vi "ErrorLog_LogError.vi"(8 "error in (no error)":errorcluster, 9 "Context (\"Error\")":string="Error", 10 "Error To Log":errorcluster, 11 "reference in":refnum<class "ErrorLog.lvclass">) -> (0 "error out":errorcluster, 1 "Error String":string, 2 "Cleaned Error":errorcluster, 3 "reference out":refnum<class "ErrorLog.lvclass">, 4 "Error was Logged":bool)   [LabVIEW 2014, in "ErrorLog.lvclass"]
uses:
  ErrorLog.lvclass
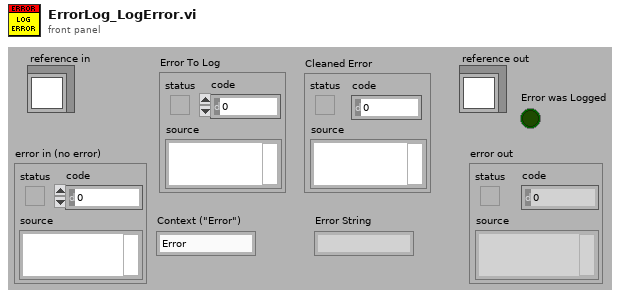
[diagram p1: front panel]
types:
  T1 = typedef "ErrorLog.lvclass/ObjectAttributes.ctl" = cluster{"ErrorFile":path, "Supress Consecutive Duplicates":bool, "Errors":string, "Quit":bool, "Errors since last call":string, "Last Recorded Error":string, "ErrorPath":path, "PossiblePaths":path[], "BaseFileName":string, "Max Log Files":i32, "ErrorFile Index":i32, "Max File Size":i64}
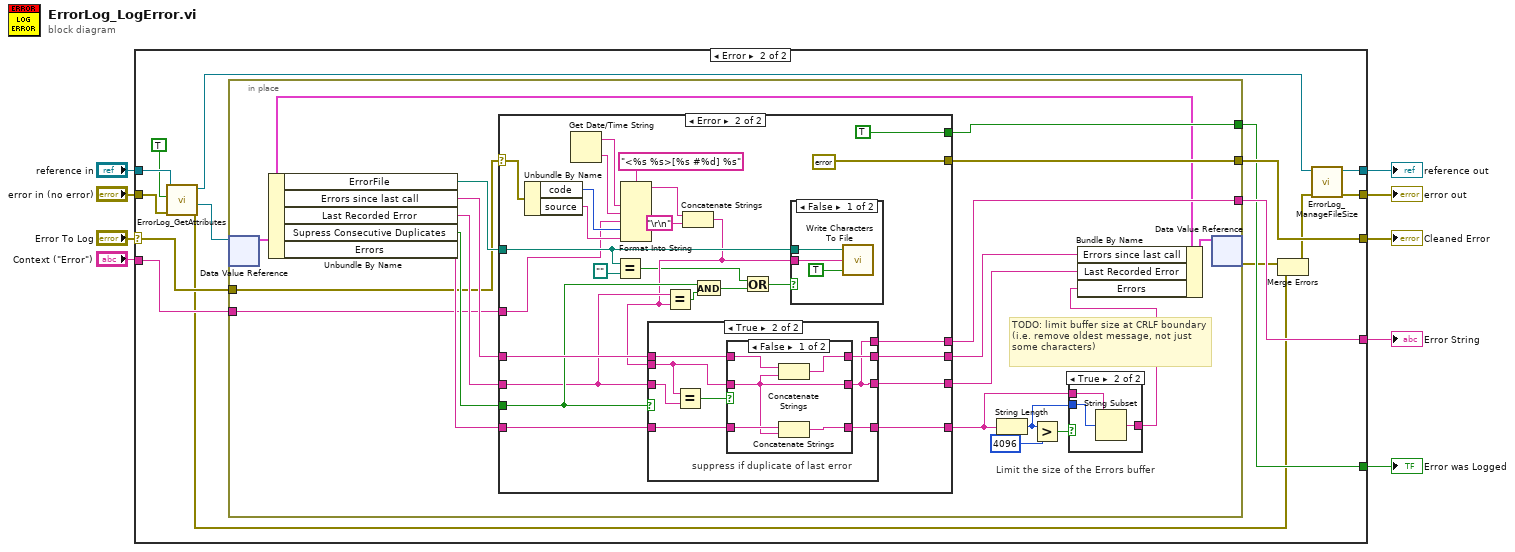
[diagram p0: block diagram]
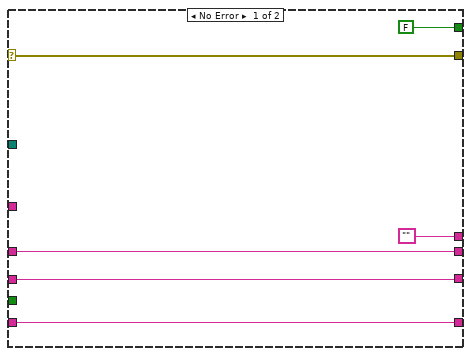
[diagram p4: hidden frame]
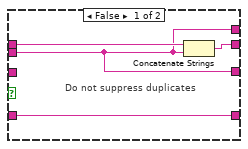
[diagram p6: hidden frame]
diagram:
  n1 = case shown="Error" "Error To Log" {
    selector: "Error To Log" -> [w11 w19]
    tunnel: [w11 w15] -> w9
    tunnel: [w10 w12] -> w7
    tunnel: "reference in" -> [w10 w26]
    tunnel: [_ w21] -> w6
    tunnel: [_ w23] -> w5
    tunnel: "error in (no error)" -> [_ w25]
    tunnel: "Context (\"Error\")" -> [_ w18]
    tunnel: [_ w22] -> w1
    frame No Error {
    }
    frame Error {
      n2 = call "ErrorLog_GetAttributes.vi"("error in (no error)"=w25, "OnlyGetDvrReference(False)"=TRUE, "reference in"=w26) -> ("error out"=w16:errorcluster, "DataRef"=w20:refnum<data-value>, "reference out"=w13:refnum<class "ErrorLog.lvclass">)  [unwired: 5 in, 1 out]
      n3 = in-place {
        in-place-border: [w33] -> w23
        in-place-border: [w32] -> w22
        in-place-border: [w31] -> w21
        in-place-border: w19 -> [w28]
        in-place-border: w18 -> [w27]
        # "TODO: limit buffer size at CRLF boundary (i.e. remove oldest message, not just some characters)"
        # "Limit the size of the Errors buffer"
        n4 = in-place-dvr #1(w20) -> (w30:T1)  [unwired: 1 out]
        n5 = Unbundle By Name(w30) -> ("ErrorFile"=w45:path, "Errors since last call"=w44:string, "Last Recorded Error"=w43:string, "Supress Consecutive Duplicates"=w42:bool, "Errors"=w39:string)
        n6 = case shown="Error" w28 {
          selector: w28 -> [w55 w80]
          tunnel: [w55 errorcluster {"status"=FALSE, "code"=0, "source"=""} ("error out")] -> w33
          tunnel: w45 -> [_ w67]
          tunnel: w44 -> [w54 w72]
          tunnel: [w54 w71] -> w40
          tunnel: w43 -> [w53 w64]
          tunnel: w42 -> [_ w65]
          tunnel: [w53 w70] -> w41
          tunnel: ["" w69] -> w32
          tunnel: [FALSE TRUE] -> w31
          tunnel: w39 -> [w50 w58]
          tunnel: [w50 w57] -> w35
          tunnel: w27 -> [_ w56]
          frame No Error {
          }
          frame Error {
            n7 = Unbundle By Name(w80) -> ("code"=w75:i32, "source"=w76:string)
            n8 = Get Date/Time String() -> (date string=w73:string, time string=w74:string)  [unwired: 3 in]
            n9 = Equal?(x=w67, y=path "") -> (x = y?=w61:bool)
            n10 = Format Into String(format string="<%s %s>[%s #%d] %s", w73, w74, w56, w75, w76) -> (resulting string=w77:string)  [unwired: 2 in, 1 out]
            n11 = Concatenate Strings(w77, "\r\n") -> (w63:string)
            n12 = case shown="True" w65 {
              tunnel: w72 -> [w88 w94]
              tunnel: w63 -> [w86 w92]
              tunnel: [w87 w93] -> w71
              tunnel: w64 -> [_ w95]
              tunnel: [w86 w91] -> w70
              tunnel: [w86 w91] -> w69
              tunnel: w58 -> [w85 w90]
              tunnel: [w85 w89] -> w57
              frame False {
                # "Do not suppress duplicates"
                n13 = Concatenate Strings(w88, w86) -> (w87:string)
              }
              frame True {
                # "suppress if duplicate of last error"
                n14 = Equal?(x=w92, y=w95) -> (x = y?=w96:bool)
                n15 = case shown="False" w96 {
                  tunnel: w92 -> [w98 w103]
                  tunnel: w94 -> [w101 w104]
                  tunnel: [w100 w104] -> w93
                  tunnel: [w98 w103] -> w91
                  tunnel: w90 -> [w99 w102]
                  tunnel: [w97 w102] -> w89
                  frame False {
                    n16 = Concatenate Strings(w101, w98) -> (w100:string)
                    n17 = Concatenate Strings(w99, w98) -> (w97:string)
                  }
                  frame True {
                    # "do not record again"
                  }
                }
              }
            }
            n18 = Equal?(x=w64, y=w63) -> (x = y?=w66:bool)
            n19 = And(x=w65, y=w66) -> (x .and. y?=w62:bool)
            n20 = Or(x=w61, y=w62) -> (x .or. y?=w60:bool)
            n21 = case shown="False" w60 {
              tunnel: w63 -> [w83 _]
              tunnel: w67 -> [w82 _]
              frame False {
                n22 = call <vilib>:"Write Characters To File.vi"("append to file? (new file:F)"=TRUE, "character string"=w83, "file path (dialog if empty)"=w82) -> ()  [unwired: 2 in, 1 out]
              }
              frame True {
                # "Object may already be destroyed"
                # "No File or suppressed"
              }
            }
          }
        }
        n23 = String Length(string=w35) -> (length=w36:i32)
        n24 = Greater?(x=w36, y=4096) -> (0:w37:bool)
        n25 = case shown="True" w37 {
          tunnel: w36 -> [_ w49]
          tunnel: w35 -> [w46 w48]
          tunnel: [w46 w47] -> w34
          frame False {
          }
          frame True {
            n26 = String Subset(string=w48, offset (0)=w49) -> (substring=w47:string)  [unwired: 1 in]
          }
        }
        n27 = Bundle By Name(cluster=w30, "Errors since last call"=w40, "Last Recorded Error"=w41, "Errors"=w34) -> (w29:T1)
        n28 = in-place-dvr #1(w29) -> (w17:errorcluster)  [unwired: 1 out]
      }
      n29 = Merge Errors(w17, w16) -> (w14:errorcluster)
      n30 = call-dynamic "ErrorLog_ManageFileSize.vi"("error in (no error)"=w14, "reference in"=w13) -> ("error out"=w15:errorcluster, "reference out"=w12:refnum<class "ErrorLog.lvclass">)  [unwired: 8 in]
    }
  }
  "error out" <- w9
  "reference out" <- w7
  "Cleaned Error" <- w5
  "Error was Logged" <- w6
  "Error String" <- w1
